vi "Read Data Block.vi"(8 "error in (no error)":errorcluster, 11 "Modicon PLC in":refnum<class "MB PLC Client.lvclass">) -> (0 "error out":errorcluster, 2 "Data Block":refnum<class "MB Data Block.lvclass">, 3 "Modicon PLC out":refnum<class "MB PLC Client.lvclass">)   [LabVIEW 2018, in "MB PLC Client.lvlib" / "MB PLC Client.lvclass"]
uses:
  MB PLC Client.lvclass
  Data/MB Data Block.lvclass
  MB PLC Client.lvclass/MB PLC Client.ctl
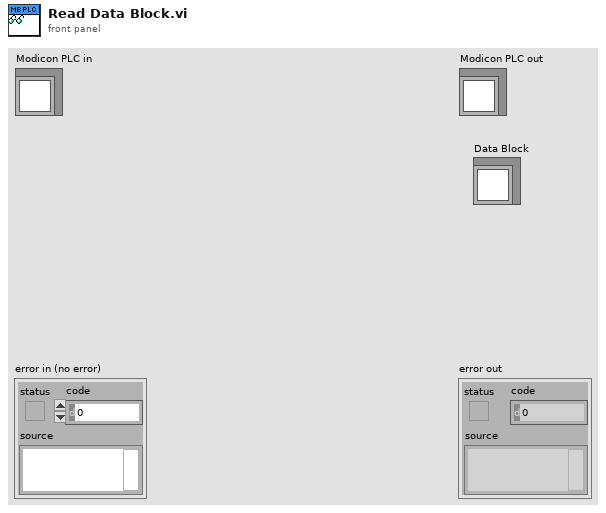
[diagram p1: front panel]
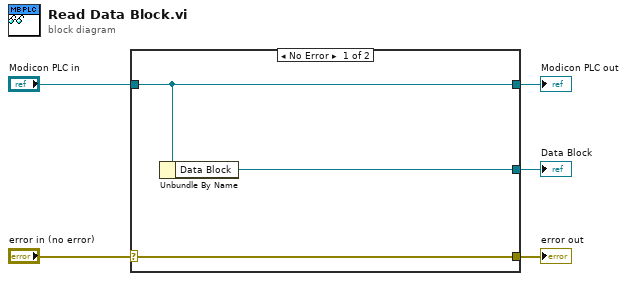
[diagram p0: block diagram]
diagram:
  n1 = case shown="No Error" "error in (no error)" {
    selector: "error in (no error)" -> [w8 w9]
    tunnel: [w8 w9] -> w4
    tunnel: [w7 w10] -> w2
    tunnel: "Modicon PLC in" -> [w7 w10]
    tunnel: [w6 _] -> w1
    frame No Error {
      n2 = Unbundle By Name(w7) -> ("Data Block"=w6:refnum<class "MB Data Block.lvclass">)
    }
    frame Error {
    }
  }
  "error out" <- w4
  "Modicon PLC out" <- w2
  "Data Block" <- w1
